vi "Pump Action-Status Analog Output.vi"(8 "error in (no error)":errorcluster, 10 "Message Data":variant, 11 "Data Cluster in":T1 {"Pump Info"."Direction" items=["CW", "CCW"]; "Pump Info"."Speed" format="%03.0f"}) -> (0 "error out":errorcluster, 3 "Data Cluster out":T1 {"Pump Info"."Direction" items=["CW", "CCW"]; "Pump Info"."Speed" format="%03.0f"})   [LabVIEW 2020, in "Pump.lvlib"]
uses:
  Pump.lvlib
  Pump Hardware Configuration.ctl
  support/Message Queue/Message Cluster.ctl
  support/HW Message Cluster.ctl
  support/Message Queue/Message Queue.lvlib
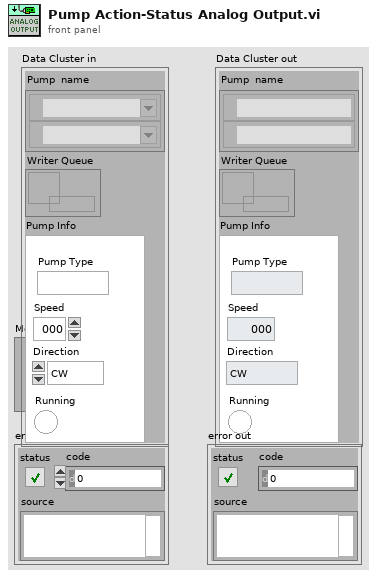
[diagram p1: front panel]
types:
  T1 = typedef "Pump.lvlib/Pump Hardware Configuration.ctl" = cluster{"Pump  name":refnum<visa-resource-name>[], "Writer Queue":refnum<queue>, "Pump Info":cluster{"Pump Type":string, "Speed":i32, "Direction":u16, "Running":bool}}
  T2 = typedef "Message Queue.lvlib/HW Message Cluster.ctl" = cluster{"Writer Queue":refnum<queue>, "Writer Data":T3}
  T3 = typedef "Message Queue.lvlib/Message Cluster.ctl" = cluster{"Message":string, "Message Data":variant}
  T4 = cluster{"Analog Output (F:1)":bool, "Slot Number (1)":i32, "Set/Check (F:Set)":bool, "Voltage (0)":dbl}
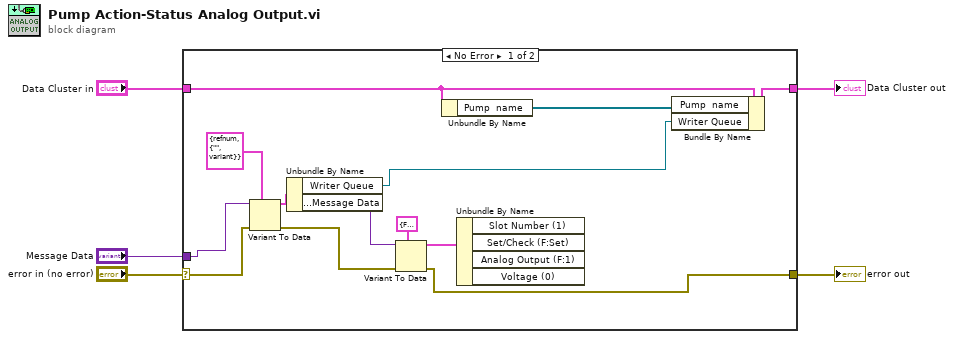
[diagram p0: block diagram]
diagram:
  n1 = case shown="No Error" "error in (no error)" {
    selector: "error in (no error)" -> [w11 w19]
    tunnel: "Message Data" -> [w9 _]
    tunnel: [w16 w20] -> w4
    tunnel: "Data Cluster in" -> [w15 w20]
    tunnel: [w18 w19] -> w2
    frame No Error {
      n2 = Variant To Data(error in=w11, type=T2 {"Writer Queue"=refnum, "Writer Data"={"Message"="", "Message Data"=variant}}, Variant=w9) -> (data=w12:T2, error out=w10:errorcluster)
      n3 = Unbundle By Name(w12) -> ("Writer Queue"=w7:refnum<queue>, "Writer Data.Message Data"=w8:variant)
      n4 = Variant To Data(error in=w10, type=T4 {"Analog Output (F:1)"=FALSE, "Slot Number (1)"=1, "Set/Check (F:Set)"=FALSE, "Voltage (0)"=0.0}, Variant=w8) -> (data=w13:T4, error out=w18:errorcluster)
      n5 = Unbundle By Name(w15) -> ("Pump  name"=w17:refnum<visa-resource-name>[])
      n6 = Unbundle By Name(w13) -> ()  [unwired: 4 out]
      n7 = Bundle By Name(cluster=w15, "Pump  name"=w17, "Writer Queue"=w7) -> (w16:T1)
    }
    frame Error {
    }
  }
  "Data Cluster out" <- w4
  "error out" <- w2
